vi "_DServerStop.vi"(2 "error in":errorcluster, 3 "dserver evt.":T1) -> (0 "error out":errorcluster)   [LabVIEW 2014, in "tango.lvlib"]
uses:
  tango.lvlib
  tango_binding.so
  Client Request Handling/Typedefs/_DServerClientRequestType.ctl
  Private VIs/Typedefs/_GenericDataBuffer.ctl
  Client Request Handling/Typedefs/_DServerClientRequestData.ctl
  Client Request Handling/Typedefs/_DServerClientRequest.ctl
  Client Request Handling/Typedefs/_DServerEvent.ctl
  Common VIs/Typedefs/_AttributeDataType_t.ctl
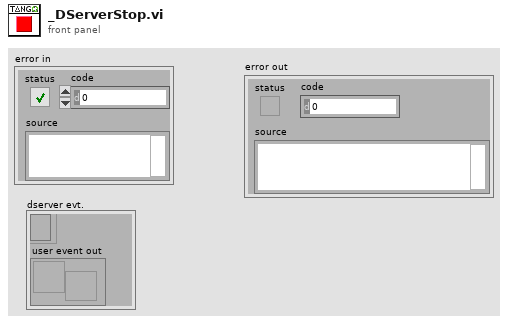
[diagram p1: front panel]
types:
  T1 = typedef "tango.lvlib/_DServerEvent.ctl" = cluster{"event registration refnum":refnum<event-registration>, "user event out":refnum<user-event>}
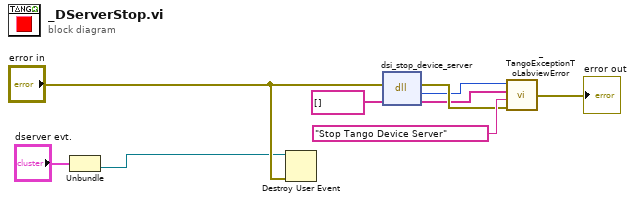
[diagram p0: block diagram]
diagram:
  n1 = Unbundle("dserver evt.") -> ("user event out"=w1:refnum<user-event>)  [unwired: 1 out]
  n2 = Destroy User Event(user event=w1, error in="error in") -> ()  [unwired: 1 out]
  n3 = dll-call lib="tango_binding.*" fn="dsi_stop_device_server"(error in="error in", "error_stack"=string[] [] ("error stack")) -> (error out=w8:errorcluster, "return type"=w6:i32, "error_stack"=w5:string[])  [unwired: 2 in, 1 out]
  n4 = call "_TangoExceptionToLabviewError.vi"("error in"=w8, "location"="Stop Tango Device Server", "error stack"=w5, "error code"=w6) -> ("error out"=→"error out":errorcluster)
